vi "duration_to_postgres_interval.vi"(8 "error in (no error)":errorcluster, 11 "relative_time":dbl) -> (0 "error out":errorcluster, 3 "interval":string)   [LabVIEW 2015, in "lv-timescaledb.lvlib"]
uses:
  lv-timescaledb.lvlib
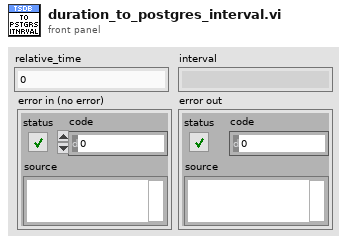
[diagram p1: front panel]
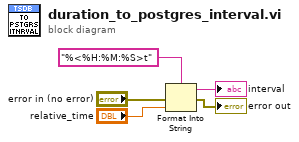
[diagram p0: block diagram]
diagram:
  n1 = Format Into String(format string="%<%H:%M:%S>t", error in="error in (no error)", "relative_time") -> (resulting string=→"interval":string, error out=→"error out":errorcluster)  [unwired: 1 in]
